vi "Count Strings.vi"(11 "strings in":T1) -> (3 "count":i32)   [LabVIEW 2023]
uses:
  <extravilib>/ChannelInstances/Stream-str/)Channel.ctl
  <extravilib>/ChannelInstances/Stream-str/Read With Abort.vi
  <extravilib>/ChannelInstances/Stream-str/EndpointRead.vi
  <extravilib>/ChannelInstances/Stream-str/)Channel.vi
  <resource>/ChannelSupport/_ChannelSupport/WaitIfNeeded.vi
  <extravilib>/ChannelInstances/Stream-str.lvlib
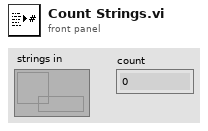
[diagram p1: front panel]
types:
  T1 = typedef "Stream-str.lvlib/)Channel.ctl" = refnum<queue>
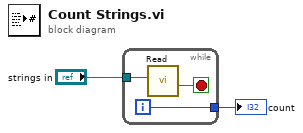
[diagram p0: block diagram]
diagram:
  n1 = while {
    tunnel: [w5] -> w2
    tunnel: "strings in" -> [w4]
    i -> [w5]
    stop <- w3 stop-if-true
    n2 = call <extravilib>:"Read.vi"("channel"=w4) -> ("last element?"=w3:bool)  [unwired: 6 in, 4 out]
  }
  "count" <- w2
